vi "writeToXML.vi"(8 "error in (no error)":errorcluster, 10 "ClassLabel":string, 11 "MccStop in":refnum<class "MccStop.lvclass">) -> (0 "error out":errorcluster, 2 "XMLout":string, 3 "MccStop out":refnum<class "MccStop.lvclass">)   [LabVIEW 2014, in "TCSDataDefinitions.lvlib" / "TCSMountControlCommand.lvlib" / "CommandsForAllAxes.lvlib" / "MccStop.lvclass"]
uses:
  MccStop.lvclass
  CommandsForAllAxes.lvclass
  <userlib>/Common/XML/XMLGenerator/XMLGenerator.lvclass
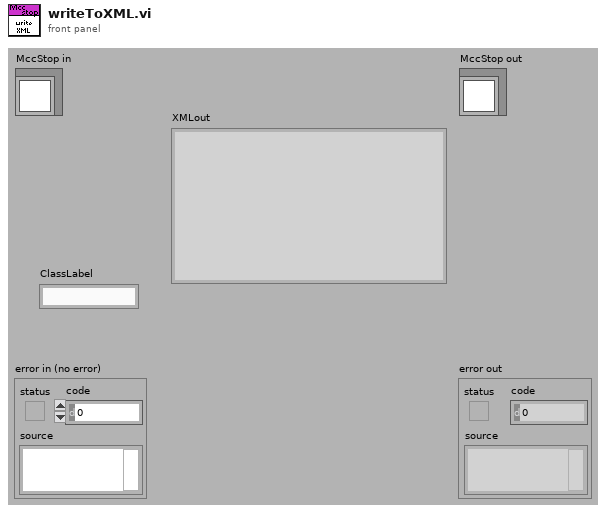
[diagram p1: front panel]
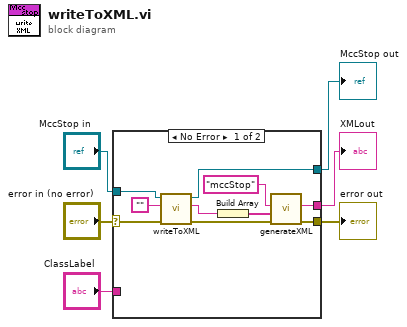
[diagram p0: block diagram]
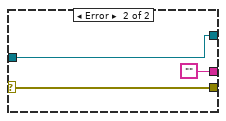
[diagram p2: hidden frame]
diagram:
  n1 = case shown="No Error" "error in (no error)" {
    selector: "error in (no error)" -> [w8 w19]
    tunnel: [w7 w19] -> w5
    tunnel: [w10 w18] -> w3
    tunnel: "MccStop in" -> [w11 w18]
    tunnel: [w9 ""] -> w2
    tunnel: "ClassLabel" -> [_ _]
    frame No Error {
      n2 = call-parent "writeToXML.vi"("error in (no error)"=w8, "ClassLabel"="", "CommandsForAllAxes in"=w11) -> ("error out"=w12:errorcluster, "XMLout"=w15:string, "CommandsForAllAxes out"=w10:refnum<class "MccStop.lvclass">)  [unwired: 6 in]
      n3 = Build Array(w15) -> (w14:string[])
      n4 = call <userlib>:"generateXML.vi"("error in"=w12, "childrenXML"=w14, "elementName"="mccStop" ("Class Label")) -> ("error out"=w7:errorcluster, "XML out"=w9:string)  [unwired: 6 in, 1 out]
    }
    frame Error {
    }
  }
  "error out" <- w5
  "MccStop out" <- w3
  "XMLout" <- w2
